vi "RF_Synth_query.vi"(2 "write buffer":string, 3 "VISA resource name":refnum<visa-resource-name>="COM8") -> (0 "error?":bool, 1 "read buffer":string)   [LabVIEW 2013]
uses:
  <vilib>/Utility/error.llb/DialogType.ctl
  <vilib>/Instr/_visa.llb/VISA Configure Serial Port (Instr).vi
panel:
  out "#bytes to read":u32
  out "Waiting\nResponse":bool
  in  "flow control":u16(ring) items=["None"=0, "XON/XOFF"=1, "RTS/CTS"=2, "DTR/DSR"=4]
  in  "stop bits":u16(ring)=10 items=["1.0"=10, "1.5"=15, "2.0"=20]
  in  "parity":u16(ring) items=["None", "Odd", "Even", "Mark", "Space"]
  in  "data bits":u16=8 min=5 max=8 step=1
  in  "baud rate":u32=115200
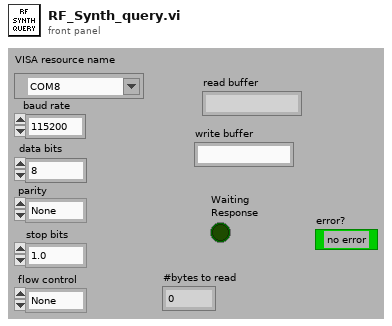
[diagram p1: front panel]
types:
  T1 = typedef "DialogType.ctl" = u16
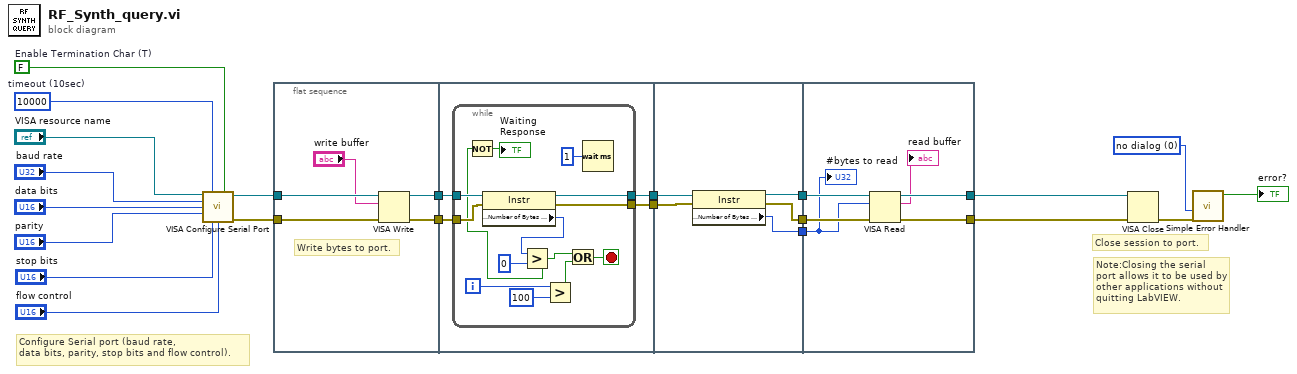
[diagram p0: block diagram]
diagram:
  w2 = T1 0 items=["no dialog", "OK message", "continue or stop message", "OK message + warnings", "continue/stop + warnings"] ("type of dialog (OK msg:1)")
  w8 = FALSE  # Enable Termination Char (T)
  w9 = u32 10000  # timeout (10sec)
  # "Note:Closing the serial port allows it to be used by other applications without\nquitting LabVIEW."
  # "Configure Serial port (baud rate,\ndata bits, parity, stop bits and flow control)."
  # "Close session to port."
  n1 = call-poly "VISA Configure Serial Port"("VISA resource name"="VISA resource name", "timeout (10sec)"=w9, "Enable Termination\nChar (T)"=w8, "baud rate (9600)"="baud rate", "data bits (8)"="data bits", "parity (0:none)"="parity", "stop bits (10: 1 bit)"="stop bits", "flow control (0:none)"="flow control") -> ("VISA resource name out"=w12:refnum<visa-resource-name>, "error out"=w13:errorcluster)  [unwired: 1 in, 5 out]
  n2 = flat-sequence {
    tunnel: w13 -> [w27]
    tunnel: w12 -> [w26]
    tunnel: [w25] -> w22
    tunnel: [w24] -> w21
    tunnel: w22 -> [w31]
    tunnel: [w30] -> w20
    tunnel: w21 -> [w29]
    tunnel: [w28] -> w19
    tunnel: w20 -> [w49]
    tunnel: [w48] -> w18
    tunnel: w19 -> [w47]
    tunnel: [w46] -> w17
    tunnel: [w45] -> w16
    tunnel: [w53] -> w4
    tunnel: [w52] -> w3
    tunnel: w18 -> [w55]
    tunnel: w17 -> [w54]
    tunnel: w16 -> [w50]
    frame #0 {
      # "Write bytes to port."
      n3 = VISA Write(VISA resource name=w26, write buffer="write buffer", error in (no error)=w27) -> (VISA resource name out=w25:refnum<visa-resource-name>, error out=w24:errorcluster)  [unwired: 1 out]
    }
    frame #1 {
      n4 = while {
        tunnel: w31 -> [w44]
        tunnel: [w43] -> w30
        tunnel: w29 -> [w42]
        tunnel: [w41] -> w28
        i -> [w33]
        stop <- w37 stop-if-true
        n5 = property class="Instr"(reference=w44, error in=w42) -> (reference out=w43:refnum<visa-resource-name>, error out=w41:errorcluster, "Serial Settings:Number of Bytes at Serial Port"=w40:u32)
        n6 = Greater?(x=w40, y=u32 0) -> (0:w36:bool)
        n7 = Not(x=w36) -> (.not. x?=→"Waiting\nResponse":bool)
        n8 = Greater?(x=w33, y=100) -> (0:w34:bool)
        n9 = Or(x=w36, y=w34) -> (x .or. y?=w37:bool)
        n10 = Wait (ms)(milliseconds to wait=u32 1) -> ()  [unwired: 1 out]
      }
    }
    frame #2 {
      n11 = property class="Instr"(reference=w49, error in=w47) -> (reference out=w48:refnum<visa-resource-name>, error out=w46:errorcluster, "Serial Settings:Number of Bytes at Serial Port"=w45:u32)
    }
    frame #3 {
      n12 = VISA Read(VISA resource name=w55, byte count=w50, error in (no error)=w54) -> (VISA resource name out=w52:refnum<visa-resource-name>, read buffer=→"read buffer":string, error out=w53:errorcluster)  [unwired: 1 out]
      "#bytes to read" <- w50
    }
  }
  n13 = VISA Close(VISA resource name=w3, error in (no error)=w4) -> (error out=w11:errorcluster)
  n14 = call <vilib>:"Simple Error Handler.vi"("type of dialog (OK msg:1)"=w2, "error in (no error)"=w11) -> ("error?"=→"error?":bool)  [unwired: 7 out]
